vi "Zamojski_Host_C.vi"() -> ()   [LabVIEW 2020]
panel:
  out "Waveform Graph":dbl[](graph)
  in  "SEND":bool
  in  "STOP":bool
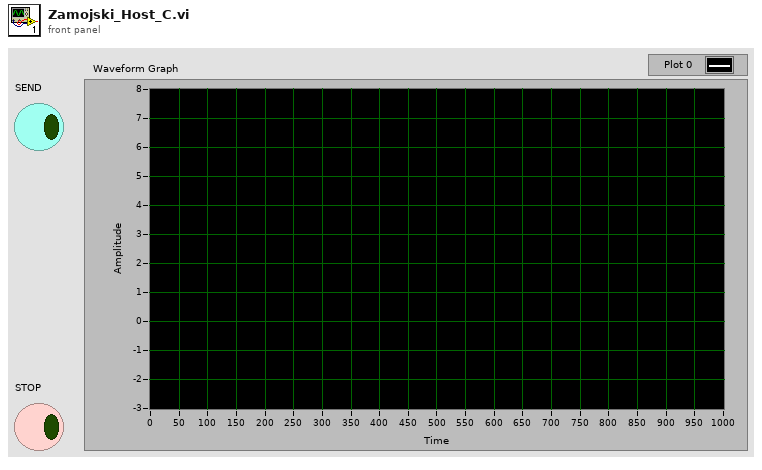
[diagram p1: front panel]
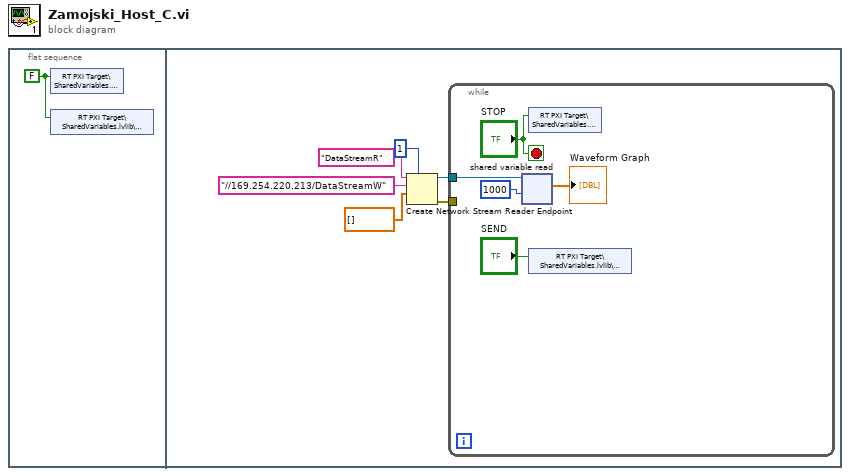
[diagram p0: block diagram]
diagram:
  n1 = flat-sequence {
    frame #0 {
      w1 = FALSE ("STOP")
      n2 = shared-variable "RT PXI Target\\SharedVariables.lvlib\\STOP"(w1) -> ()  [unwired: 1 in, 1 out]
      n3 = shared-variable "RT PXI Target\\SharedVariables.lvlib\\SignalSend"(w1) -> ()  [unwired: 1 in, 1 out]
    }
    frame #1 {
      n4 = Create Network Stream Reader Endpoint(7:1 ("reader buffer size"), 9:dbl[] [], 10:"//169.254.220.213/DataStreamW" ("writer url"), 11:"DataStreamR" ("reader name")) -> (0:w5:errorcluster, 3:w4:refnum<k21>)  [unwired: 3 in]
      n5 = while {
        tunnel: w5 -> [_]
        tunnel: w4 -> [w9]
        stop <- "STOP" stop-if-true
        n6 = shared-variable-read(w9, 1000 ("timeout ms (-1)")) -> (→"Waveform Graph":dbl[])  [unwired: 1 in, 3 out]
        n7 = shared-variable "RT PXI Target\\SharedVariables.lvlib\\STOP"("STOP") -> ()  [unwired: 1 in, 1 out]
        n8 = shared-variable "RT PXI Target\\SharedVariables.lvlib\\SignalSend"("SEND") -> ()  [unwired: 1 in, 1 out]
      }
    }
  }
